vi "Get Font.vi"(8 "error in (no error)":errorcluster, 9 "System Fonts":T1, 10 "Font IN":T2={"Name"="Helvetica", "Size"=12.0, "Color"=0, "Style"={"Bold"=FALSE, "Italic"=FALSE, "Underline"=FALSE, "Strikeout"=FALSE}}) -> (0 "error out":errorcluster, 1 "Font OUT":T2={"Name"="Helvetica", "Size"=12.0, "Color"=0, "Style"={"Bold"=FALSE, "Italic"=FALSE, "Underline"=FALSE, "Strikeout"=FALSE}}, 2 "Font Size":T3=12.0, 3 "Font":refnum<k24>)   [LabVIEW 2013]
doc: "Version 1.0\nDeveloped by Jean-Marc Simard\nCopyright © 2010, Exaprom Inc.\nAll rights reserved.\nLicense: BSD\n\nWith iTextSharp 4.1.6 (http://itextsharp.sourceforge.net)\nunder Mozilla Public License Version 1.1\n(http://www.mozilla.org/MPL/MPL-1.1.html)"
uses:
  Controls/Font cluster.ctl
  Controls/Font size.ctl
  Controls/Font color.ctl
  C:/Users/MaxCorp/Documents/GitHub/TopView/DLL/itextsharp.dll
  DLL/itextsharp.dll
  Controls/System Fonts.ctl
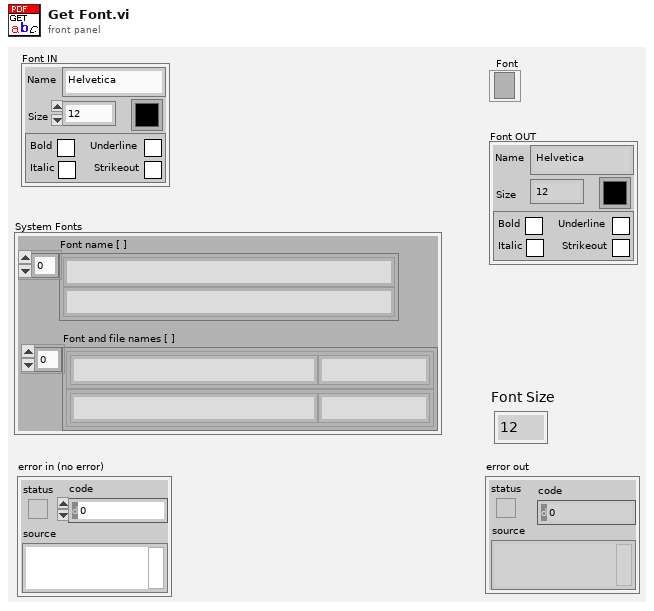
[diagram p1: front panel]
types:
  T1 = typedef "System Fonts.ctl" = cluster{"Font name [ ]":string[], "Font and file names [ ]":cluster{"Font name":string, "File name":string}[]}
  T2 = typedef "Font cluster.ctl" = cluster{"Name":string, "Size":T3, "Color":T4, "Style":cluster{"Bold":bool, "Italic":bool, "Underline":bool, "Strikeout":bool}}
  T3 = typedef "Font size.ctl" = sgl
  T4 = typedef "Font color.ctl" = u32
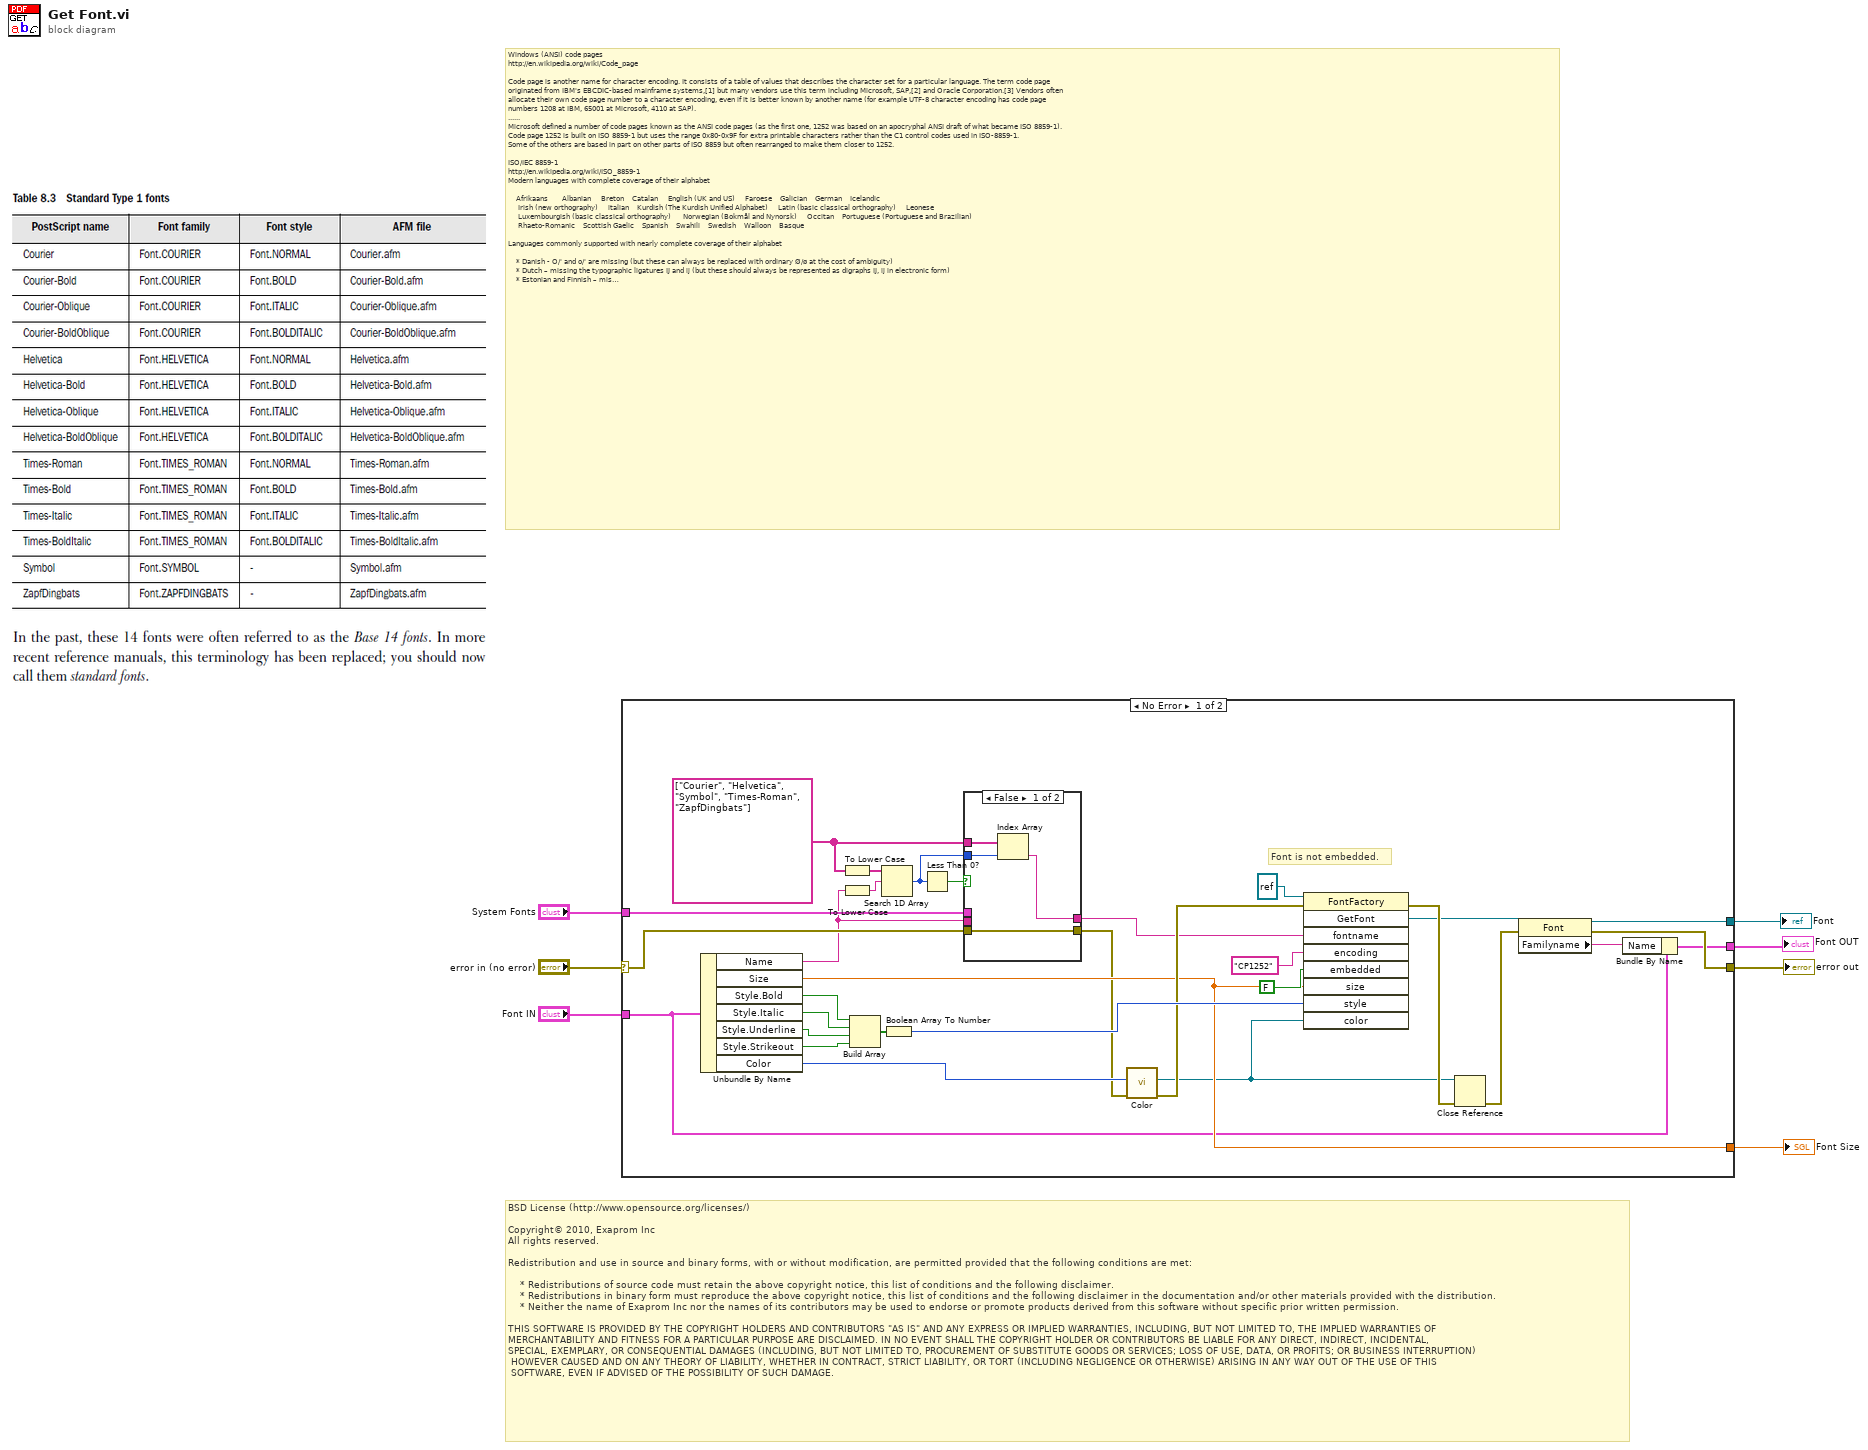
[diagram p0: block diagram]
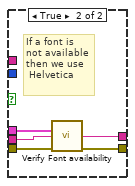
[diagram p2: hidden frame]
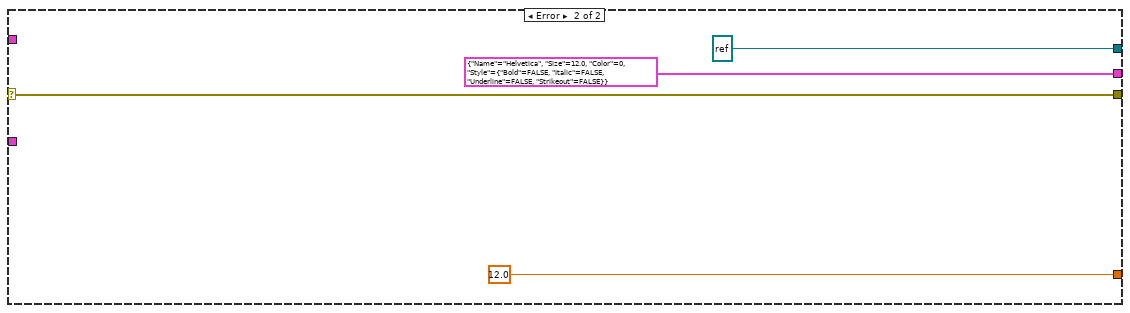
[diagram p3: hidden frame]
diagram:
  # "Windows (ANSI) code pages\nhttp://en.wikipedia.org/wiki/Code_page\n\nCode page is another name for character encoding. It consists of a table of values that describes the character set for a particular language. The term code page\noriginated from IBM's EBCDIC-based mainframe systems,[1] but many vendors use this term including Microsoft, SAP,[2] and Oracle Corporation.[3] Vendors often\nallocate their own code page number to a character encoding, even if it is better known by another name (for example UTF-8 character encoding has code page \nnumbers 1208 at IBM, 65001 at Microsoft, 4110 at SAP).\n......\nMicrosoft defined a number of code pages known as the ANSI code pages (as the first one, 1252 was based on an apocryphal ANSI draft of what became ISO 8859-1). \nCode page 1252 is built on ISO 8859-1 but uses the range 0x80-0x9F for extra printable characters rather than the C1 control codes used in ISO-8859-1. \nSome of the others are based in part on other parts of ISO 8859 but often rearranged to make them closer to 1252.\n\nISO/IEC 8859-1\nhttp://en.wikipedia.org/wiki/ISO_8859-1\nModern languages with complete coverage of their alphabet\n\n    Afrikaans       Albanian     Breton    Catalan     English (UK and US)     Faroese    Galician    German    Icelandic\n     Irish (new orthography)     italian    Kurdish (The Kurdish Unified Alphabet)     Latin (basic classical orthography)     Leonese\n     Luxembourgish (basic classical orthography)      Norwegian (Bokmål and Nynorsk)     Occitan    Portuguese (Portuguese and Brazilian)\n     Rhaeto-Romanic    Scottish Gaelic    Spanish    Swahili    Swedish    Walloon    Basque\n\nLanguages commonly supported with nearly complete coverage of their alphabet\n\n    * Danish - O/' and o/' are missing (but these can always be replaced with ordinary Ø/ø at the cost of ambiguity)\n    * Dutch – missing the typographic ligatures IJ and ij (but these should always be represented as digraphs IJ, ij in electronic form)\n    * Estonian and Finnish – missing Š, š, Ž, ž, which can only occur in loanwords (the missing characters are often replaced by digraphs Sh, sh, Zh, zh) (Windows-1252 and ISO-8859-15 do contain these)\n    * French – missing the ligatures Œ and œ as well as the very rare Ÿ (they are generally replaced by digraphs OE and oe, and Y without the diaeresis) (Windows-1252 and ISO-8859-15 do contain these)\n    * Hungarian – missing O\", o\", U\", u\"\n    * Latin (classical language written using macrons) – missing A-, a-, E-, e-, I-, i-, O-, o-, U-, u-\n    * Welsh – missing W^, w^, Y^, y^ (ISO-8859-14 does contain these)\n    * Maori – missing A-, a-, E-, e-, I-, i-, O-, o-, U-, u-"
  # "BSD License (http://www.opensource.org/licenses/)\n\nCopyright© 2010, Exaprom Inc\nAll rights reserved.\n\nRedistribution and use in source and binary forms, with or without modification, are permitted provided that the following conditions are met:\n\n    * Redistributions of source code must retain the above copyright notice, this list of conditions and the following disclaimer.\n    * Redistributions in binary form must reproduce the above copyright notice, this list of conditions and the following disclaimer in the documentation and/or other materials provided with the distribution.\n    * Neither the name of Exaprom Inc nor the names of its contributors may be used to endorse or promote products derived from this software without specific prior written permission.\n\nTHIS SOFTWARE IS PROVIDED BY THE COPYRIGHT HOLDERS AND CONTRIBUTORS \"AS IS\" AND ANY EXPRESS OR IMPLIED WARRANTIES, INCLUDING, BUT NOT LIMITED TO, THE IMPLIED WARRANTIES OF \nMERCHANTABILITY AND FITNESS FOR A PARTICULAR PURPOSE ARE DISCLAIMED. IN NO EVENT SHALL THE COPYRIGHT HOLDER OR CONTRIBUTORS BE LIABLE FOR ANY DIRECT, INDIRECT, INCIDENTAL,\nSPECIAL, EXEMPLARY, OR CONSEQUENTIAL DAMAGES (INCLUDING, BUT NOT LIMITED TO, PROCUREMENT OF SUBSTITUTE GOODS OR SERVICES; LOSS OF USE, DATA, OR PROFITS; OR BUSINESS INTERRUPTION)\n HOWEVER CAUSED AND ON ANY THEORY OF LIABILITY, WHETHER IN CONTRACT, STRICT LIABILITY, OR TORT (INCLUDING NEGLIGENCE OR OTHERWISE) ARISING IN ANY WAY OUT OF THE USE OF THIS\n SOFTWARE, EVEN IF ADVISED OF THE POSSIBILITY OF SUCH DAMAGE."
  n1 = case shown="No Error" "error in (no error)" {
    selector: "error in (no error)" -> [w13 w49]
    tunnel: [w19 refnum<k24> refnum ("GetFont")] -> w3
    tunnel: "Font IN" -> [w14 _]
    tunnel: [w21 T3 12.0 ("Size")] -> w5
    tunnel: [w38 w49] -> w4
    tunnel: [w17 T2 {"Name"="Helvetica", "Size"=12.0, "Color"=0, "Style"={"Bold"=FALSE, "Italic"=FALSE, "Underline"=FALSE, "Strikeout"=FALSE}} ("Font IN")] -> w2
    tunnel: "System Fonts" -> [w15 _]
    frame No Error {
      w9 = string[] ["Courier", "Helvetica", "Symbol", "Times-Roman", "ZapfDingbats"] ("Strings []")
      # "Font is not embedded."
      n2 = Unbundle By Name(w14) -> ("Name"=w10:string, "Size"=w21:T3, "Style.Bold"=w36:bool, "Style.Italic"=w35:bool, "Style.Underline"=w34:bool, "Style.Strikeout"=w33:bool, "Color"=w32:T4)
      n3 = To Lower Case(string=w9) -> (all lower case string=w23:string[])
      n4 = To Lower Case(string=w10) -> (all lower case string=w22:string)
      n5 = Build Array(w36, w35, w34, w33) -> (w37:bool[])
      n6 = Search 1D Array(1D array=w23, element=w22) -> (index of element=w8:i32)  [unwired: 1 in]
      n7 = Boolean Array To Number(Boolean array=w37) -> (number=w31:u32)
      n8 = Less Than 0?(x=w8) -> (x < 0?=w24:bool)
      n9 = case shown="False" w24 {
        tunnel: [w39 w46] -> w25
        tunnel: w10 -> [_ w47]
        tunnel: w15 -> [_ w45]
        tunnel: w13 -> [w42 w44]
        tunnel: [w42 w43] -> w12
        tunnel: w9 -> [w41 _]
        tunnel: w8 -> [w40 _]
        frame False {
          n10 = Index Array(array=w41, index=w40) -> (element=w39:string)
        }
        frame True {
          # "If a font is \nnot available\nthen we use\n Helvetica"
          n11 = call "Verify Font availability.vi"("System Fonts"=w45, "Font name"=w47, "error in (no error)"=w44) -> ("Font"=w46:string, "error out"=w43:errorcluster)  [unwired: 1 in, 10 out]
        }
      }
      n12 = call "Color.vi"("error in (no error)"=w12, "Color"=w32) -> ("error out"=w26:errorcluster, "Color"=w16:refnum<k24>)  [unwired: 8 out]
      n13 = invoke class="FontFactory" method="GetFont"(reference=refnum<k24> refnum, error in=w26, "fontname"=w25, "encoding"="CP1252", "embedded"=FALSE, "size"=w21, "style"=w31, "color"=w16) -> (error out=w29:errorcluster, "GetFont"=w20:refnum<k24>)  [unwired: 1 in, 7 out]
      n14 = Close Reference(reference=w16, error in (no error)=w29) -> (error out=w11:errorcluster)
      n15 = property class="Font"(reference=w20, error in=w11) -> (reference out=w19:refnum<k24>, error out=w38:errorcluster, "Familyname"=w18:string)
      n16 = Bundle By Name(cluster=w14, "Name"=w18) -> (w17:T2)
    }
    frame Error {
    }
  }
  "error out" <- w4
  "Font" <- w3
  "Font Size" <- w5
  "Font OUT" <- w2
